vi "example_02_unload_api.vi"() -> ()   [LabVIEW 2015, in "lv-dialog-interfaces.lvlib" / "v1.lvlib"]
doc: "Use this to unload the class"
uses:
  <userlib>/antonio-alexander/lv-dialog/api/v1/public/class/v1.lvclass
  <userlib>/antonio-alexander/lv-dialog/api/v1/public/_subvis/advanced/load_class-class.vi
  v1.lvlib
  <userlib>/antonio-alexander/lv-dialog/api/v1/v1.lvlib
panel:
  out "error out":errorcluster
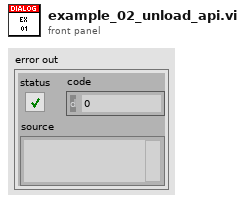
[diagram p1: front panel]
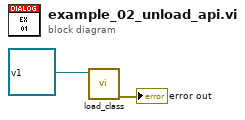
[diagram p0: block diagram]
diagram:
  n1 = call-poly <userlib>:"load_class.vi"("class"=refnum<class "v1.lvclass"> refnum) -> ("error out"=→"error out":errorcluster)  [unwired: 10 in]
